vi "Initialize.vi"(8 "error in (no error)":errorcluster, 11 "ParseGDSII in":refnum<class "ParseGDSII.lvclass">) -> (0 "error out":errorcluster, 3 "ParseGDSII out":refnum<class "ParseGDSII.lvclass">)   [LabVIEW 2020, in "ParseGDSII.lvclass"]
uses:
  ParseGDSII.lvclass
  ParseGDSII.lvclass/ParseGDSII.ctl
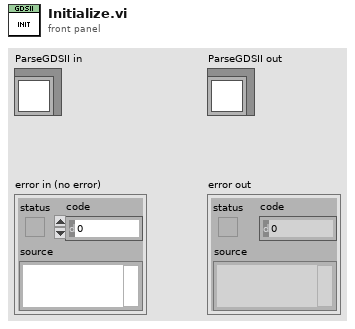
[diagram p1: front panel]
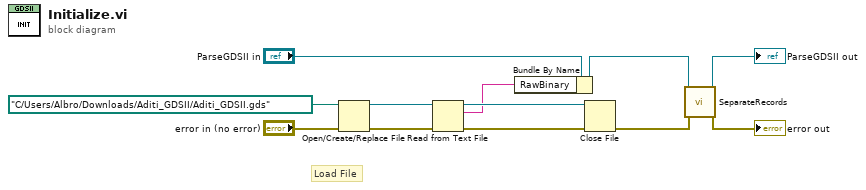
[diagram p0: block diagram]
diagram:
  # "Load File"
  n1 = Open/Create/Replace File(file path (use dialog)=path "C:/Users/Albro/Downloads/Aditi_GDSII/Aditi_GDSII.gds", error in="error in (no error)") -> (refnum out=w11:refnum<file>, error out=w9:errorcluster)  [unwired: 4 in, 1 out]
  n2 = Read from Text File(file (use dialog)=w11, error in=w9) -> (refnum out=w10:refnum<file>, text=w5:string, error out=w8:errorcluster)  [unwired: 2 in, 1 out]
  n3 = Bundle By Name(cluster="ParseGDSII in", "RawBinary"=w5) -> (w4:refnum<class "ParseGDSII.lvclass">)
  n4 = Close File(refnum=w10, error in=w8) -> (error out=w2:errorcluster)  [unwired: 1 out]
  n5 = call "SeparateRecords.vi"("error in (no error)"=w2, "ParseGDSII in"=w4) -> ("error out"=→"error out":errorcluster, "ParseGDSII out"=→"ParseGDSII out":refnum<class "ParseGDSII.lvclass">)  [unwired: 8 in]
